vi "callbackVI rising 2.vi"(11 "IRQ Number":u8) -> ()   [LabVIEW 2019]
uses:
  PING rising 1 time.vi
  <vilib>/myRIO/Common/Instrument Driver Framework/myRIO v1.0/IRQ/vis/myRIO v1.0 Reserve IRQ.vi
  <vilib>/myRIO/Common/Instrument Driver Framework/Utilities/vis/FPGA Ref Manager.vi
  <vilib>/myRIO/Common/Instrument Driver Framework/myRIO v1.0/myRIO v1.0 Close.vi
  <vilib>/myRIO/Instrument Drivers/IRQ/IO IRQ/IO IRQ.lvlib
panel:
  out "Stop?":bool
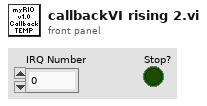
[diagram p1: front panel]
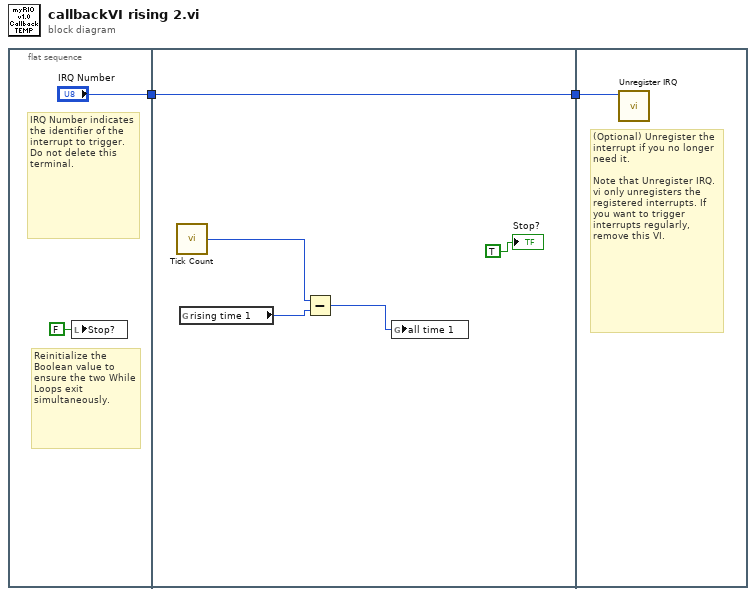
[diagram p0: block diagram]
diagram:
  n1 = flat-sequence {
    tunnel: ["IRQ Number"] -> w2
    tunnel: [w9] -> w1
    tunnel: w2 -> [w9]
    tunnel: w1 -> [w10]
    frame #0 {
      # "Reinitialize the Boolean value to ensure the two While Loops exit simultaneously."
      # "IRQ Number indicates the identifier of the interrupt to trigger. Do not delete this terminal."
      n2 = local write "Stop?"(FALSE ("Stop?")) -> ()
    }
    frame #1 {
      n3 = call "Tick Count"() -> ("Tick Count(uSec)"=w7:u32)
      n4 = global read "PING rising 1 time.vi" "rising time 1"() -> (w6:u32)
      n5 = Subtract(x=w7, y=w6) -> (x-y=w5:u32)
      n6 = global write "PING rising 1 time.vi" "all time 1"(w5) -> ()
      "Stop?" <- TRUE ("Stop?")
    }
    frame #2 {
      # "(Optional) Unregister the interrupt if you no longer need it.\n\nNote that Unregister IRQ.vi only unregisters the registered interrupts. If you want to trigger interrupts regularly, remove this VI."
      n7 = call <vilib>:"Unregister IRQ.vi"("IRQ Number"=w10) -> ()  [unwired: 10 in, 1 out]
    }
  }
